vi "dvp Vi Set Saturation.vi"(10 "Saturation":i32, 11 "handle":u32) -> (3 "function return":u32(ring))   [LabVIEW 2018, in "LabViewDVPCamera.lvlib"]
doc: "LabviewDvp2Api dvpStatus dvpViSetSaturation(dvpHandle handle, dvpInt32 Saturation);"
uses:
  LabViewDVPCamera.lvlib
  LabViewDVPCamera/LabViewDVPCamera.dll
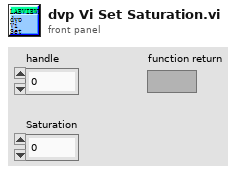
[diagram p1: front panel]
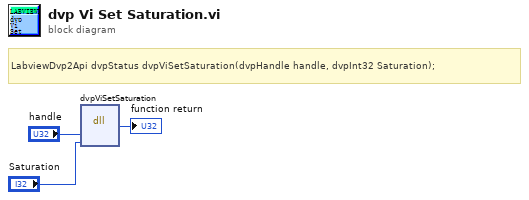
[diagram p0: block diagram]
diagram:
  # "LabviewDvp2Api dvpStatus dvpViSetSaturation(dvpHandle handle, dvpInt32 Saturation);"
  n1 = dll-call lib="C:/Program Files (x86)/DVP2 Labview cn 64/Sample/LabViewDVPCamera/LabViewDVPCamera.*" fn="dvpViSetSaturation"("handle"="handle", "Saturation"="Saturation") -> (→"function return":u32)  [unwired: 5 in, 2 out]
